vi "checkIfVIInOldLibrary.vi"(8 "error in (no error)":errorcluster, 10 "element":refnum<vi>, 11 "Dependency in":refnum<class "Dependency.lvclass">) -> (0 "error out":errorcluster, 1 "VI Path":path, 2 "isMemberOfOldLibrary":bool, 3 "Dependency out":refnum<class "Dependency.lvclass">)   [LabVIEW 2016, in "Dependency.lvclass"]
uses:
  Dependency.lvclass
  Dependency.lvclass/Dependency.ctl
  Search/Search.lvclass/Search.ctl
  Search/Search.lvclass
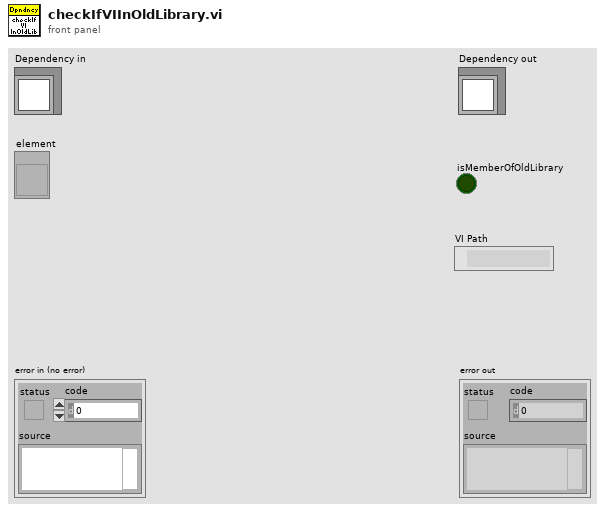
[diagram p1: front panel]
types:
  T1 = cluster{"OldLibrary":string, "NewLibrary":string}
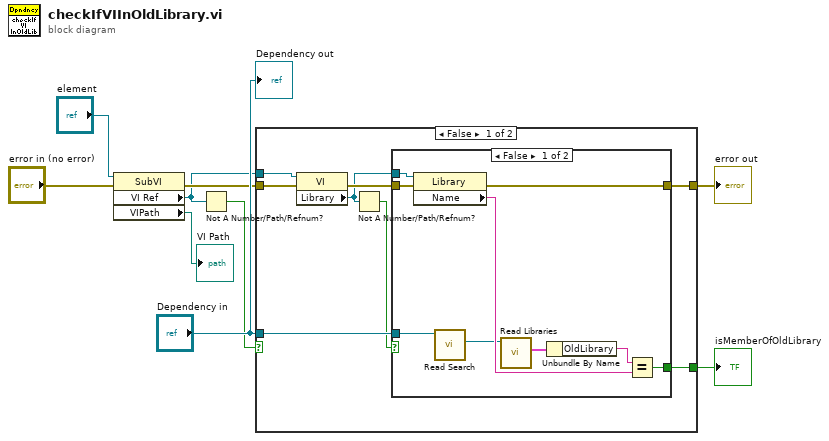
[diagram p0: block diagram]
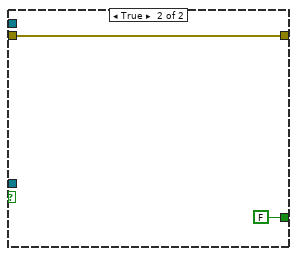
[diagram p2: hidden frame]
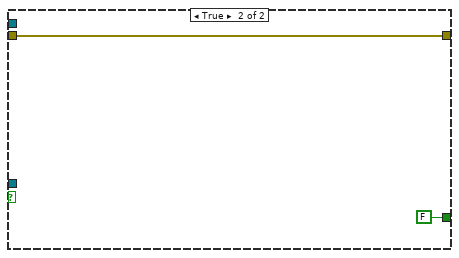
[diagram p3: hidden frame]
diagram:
  n1 = property class="SubVI"(reference="element", error in="error in (no error)") -> (error out=w5:errorcluster, "VI Ref"=w3:refnum<vi>, "VIPath"=→"VI Path":path)  [unwired: 1 out]
  n2 = Not A Number/Path/Refnum?(number/path/refnum=w3) -> (NaN/Path/Refnum?=w2:bool)
  n3 = case shown="False" w2 {
    tunnel: "Dependency in" -> [w17 _]
    tunnel: [w16 FALSE] -> w8
    tunnel: w3 -> [w15 _]
    tunnel: w5 -> [w14 w30]
    tunnel: [w12 w30] -> w4
    frame False {
      n4 = property class="VI"(reference=w15, error in=w14) -> (error out=w13:errorcluster, "Library"=w11:refnum<vi>)  [unwired: 1 out]
      n5 = Not A Number/Path/Refnum?(number/path/refnum=w11) -> (NaN/Path/Refnum?=w10:bool)
      n6 = case shown="False" w10 {
        tunnel: w17 -> [w20 _]
        tunnel: [w24 FALSE] -> w16
        tunnel: w13 -> [w23 w27]
        tunnel: [w22 w27] -> w12
        tunnel: w11 -> [w21 _]
        frame False {
          n7 = property class="Library"(reference=w21, error in=w23) -> (error out=w22:errorcluster, "Name"=w25:string)  [unwired: 1 out]
          n8 = call "Read Search.vi"("Dependency in"=w20) -> ("Search"=w19:refnum<class "Search.lvclass">)  [unwired: 9 in, 1 out]
          n9 = call "Read Libraries.vi"("ProjectItem in"=w19) -> ("Libraries"=w18:T1)  [unwired: 9 in, 1 out]
          n10 = Unbundle By Name(w18) -> ("OldLibrary"=w26:string)
          n11 = Equal?(x=w26, y=w25) -> (x = y?=w24:bool)
        }
        frame True {
        }
      }
    }
    frame True {
    }
  }
  "error out" <- w4
  "isMemberOfOldLibrary" <- w8
  "Dependency out" <- "Dependency in"
